vi "Handle INVOCATION.vi"(8 "error in (no error)":errorcluster, 9 "Message Loop Shift Register Data":T1, 10 "Cluster":T8 {"Message Codes" items=["HELLO"=1, "WELCOME"=2, "ABORT"=3, "GOODBYE"=6, "ERROR"=8, "PUBLISH"=16, "PUBLISHED"=17, "SUBSCRIBE"=32, "SUBSCRIBED"=33, "UNSUBSCRIBE"=34, "UNSUBSCRIBED"=35, "EVENT"=36, "CALL"=48, "RESULT"=59, "REGISTER"=64, "REGISTERED"=65, "UNREGISTER"=66, "UNREGISTERED"=67, "INVOCATION"=68, "YIELD"=70]}, 11 "reference":refnum<class "WAMP Client.lvclass">) -> (0 "error out":errorcluster, 3 "reference out":refnum<class "WAMP Client.lvclass">)   [LabVIEW 2020, in "wamplv.lvlib" / "WAMP Client.lvclass"]
uses:
  <userlib>/wamplv/WAMP Client/WAMP Client.lvclass
  <userlib>/wamplv/WAMP Client/TypeDef/WAMP Received Message.ctl
  <userlib>/wamplv/WAMP Message Codes.ctl
  <userlib>/wamplv/WAMP Client/TypeDef/Message Loop Shift Reg Data.ctl
  <userlib>/wamplv/WAMP Client/TypeDef/REGISTER Request Data.ctl
  <userlib>/wamplv/WAMP Client/TypeDef/REGISTERED or ERROR payload.ctl
  <userlib>/wamplv/WAMP Client/TypeDef/WAMP Error Payload.ctl
  <userlib>/wamplv/WAMP Client/TypeDef/INVOCATION payload.ctl
  <userlib>/wamplv/WAMP Client/TypeDef/Publish Requests Map.ctl
  <userlib>/wamplv/WAMP Client/TypeDef/PUBLISH Request Data.ctl
  <userlib>/wamplv/WAMP Client/TypeDef/PUBLISH Result.ctl
  <userlib>/wamplv/WAMP Client/TypeDef/Endpoint Data.ctl
  <userlib>/wamplv/WAMP Client/TypeDef/CALL Request Map.ctl
  <userlib>/wamplv/WAMP Client/TypeDef/CALL Request Data.ctl
  <userlib>/wamplv/WAMP Client/TypeDef/RESULT Payload.ctl
  <userlib>/wamplv/WAMP Client/WAMP Client.lvclass/WAMP Client.ctl
  <vilib>/JDP Science/JSONtext/JSONtext.lvlib
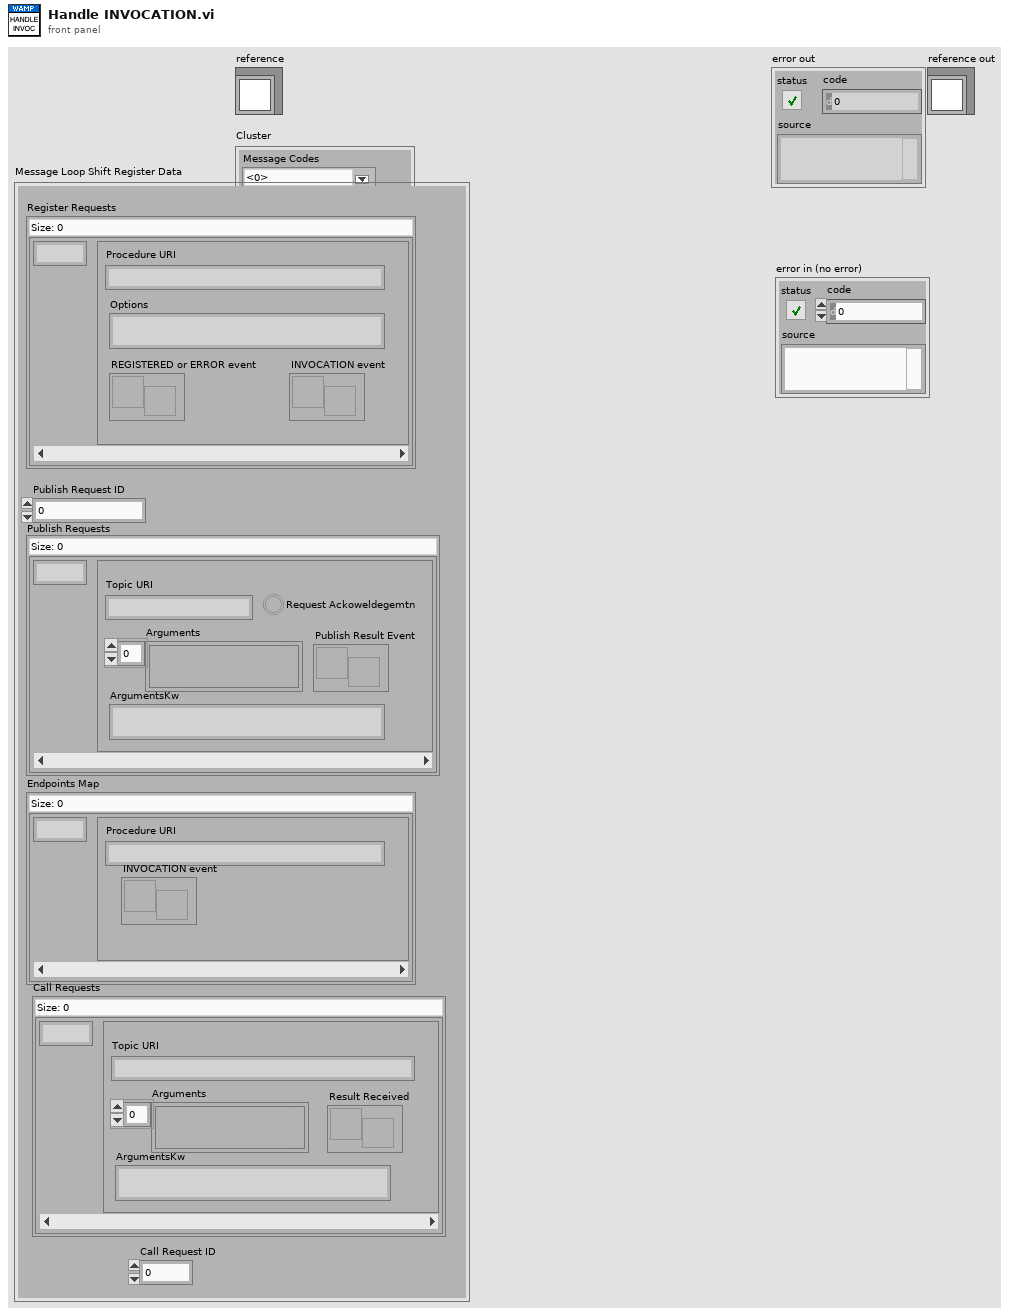
[diagram p1: front panel]
types:
  T1 = typedef "wamplv.lvlib/WAMP Client.lvclass/Message Loop Shift Reg Data.ctl" = cluster{"Register Requests":map{u32, T2}, "Publish Request ID":u32, "Publish Requests":T3, "Endpoints Map":map{u32, T5}, "Call Requests":T6, "Call Request ID":u32}
  T2 = typedef "wamplv.lvlib/WAMP Client.lvclass/REGISTER Request Data.ctl" = cluster{"Procedure URI":string, "Options":string, "REGISTERED or ERROR event":refnum<user-event>, "INVOCATION event":refnum<user-event>}
  T3 = typedef "wamplv.lvlib/WAMP Client.lvclass/Publish Requests Map.ctl" = map{u32, T4}
  T4 = typedef "wamplv.lvlib/WAMP Client.lvclass/PUBLISH Request Data.ctl" = cluster{"Topic URI":string, "Arguments":variant[], "ArgumentsKw":string, "Publish Result Event":refnum<user-event>, "Request Ackoweldegemtn":bool}
  T5 = typedef "wamplv.lvlib/WAMP Client.lvclass/Endpoint Data.ctl" = cluster{"Procedure URI":string, "INVOCATION event":refnum<user-event>}
  T6 = typedef "wamplv.lvlib/WAMP Client.lvclass/CALL Request Map.ctl" = map{u32, T7}
  T7 = typedef "wamplv.lvlib/WAMP Client.lvclass/CALL Request Data.ctl" = cluster{"Topic URI":string, "Arguments":variant[], "ArgumentsKw":string, "Result Received":refnum<user-event>}
  T8 = typedef "wamplv.lvlib/WAMP Client.lvclass/WAMP Received Message.ctl" = cluster{"Message JSON":string[], "Message Codes":T9}
  T9 = typedef "wamplv.lvlib/WAMP Client.lvclass/WAMP Message Codes.ctl" = u16
  T10 = typedef "wamplv.lvlib/WAMP Client.lvclass/INVOCATION payload.ctl" = cluster{"Arguments":string[], "ArgumentKw":string, "Procedure URI":string, "Details":string, "Registration ID":u32, "Request ID":u32}
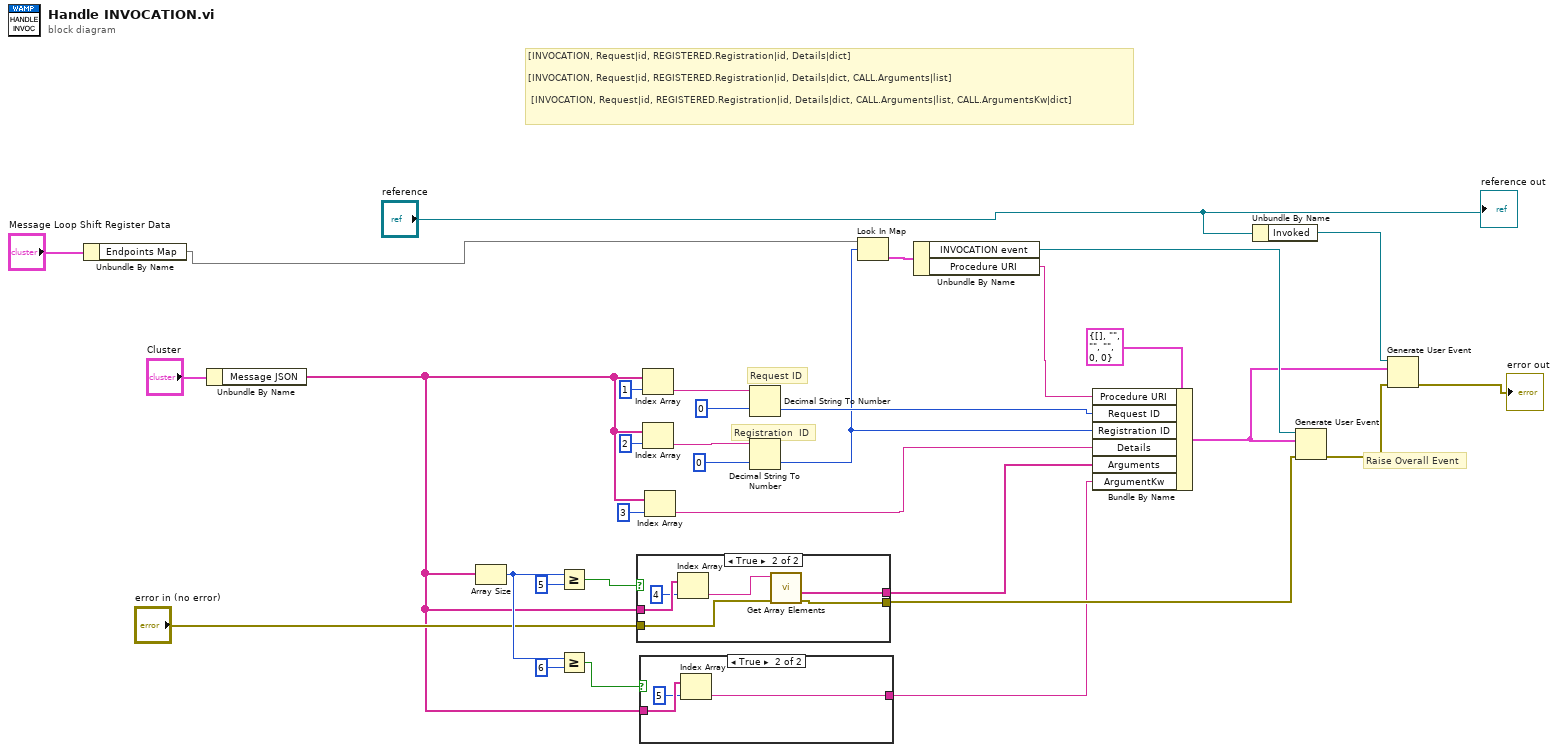
[diagram p0: block diagram]
diagram:
  # "Raise Overall Event"
  # "[INVOCATION, Request|id, REGISTERED.Registration|id, Details|dict]\n\n[INVOCATION, Request|id, REGISTERED.Registration|id, Details|dict, CALL.Arguments|list]\n\n [INVOCATION, Request|id, REGISTERED.Registration|id, Details|dict, CALL.Arguments|list, CALL.ArgumentsKw|dict]"
  # "Registration  ID"
  # "Request ID"
  n1 = Unbundle By Name("Message Loop Shift Register Data") -> ("Endpoints Map"=w10:map{u32, T5})
  n2 = Unbundle By Name("Cluster") -> ("Message JSON"=w4:string[])
  n3 = Array Size(array=w4) -> (size(s)=w22:i32)
  n4 = Greater Or Equal?(x=w22, y=5) -> (x >= y?=w24:bool)
  n5 = Greater Or Equal?(x=w22, y=6) -> (x >= y?=w21:bool)
  n6 = case shown="True" w24 {
    tunnel: w4 -> [_ w38]
    tunnel: [_ w36] -> w6
    tunnel: "error in (no error)" -> [w33 w35]
    tunnel: [w33 w34] -> w19
    frame False {
    }
    frame True {
      n7 = Index Array(array=w38, index=4) -> (element=w39:string)
      n8 = call <vilib>:"Get Array Elements.vi"("error in (no error)"=w35, "JSON"=w39) -> ("error out"=w34:errorcluster, "<JSON>"=w36:string[])  [unwired: 7 in, 1 out]
    }
  }
  n9 = case shown="True" w21 {
    tunnel: w4 -> [_ w42]
    tunnel: [_ w40] -> w5
    frame False {
    }
    frame True {
      n10 = Index Array(array=w42, index=5) -> (element=w40:string)
    }
  }
  n11 = Index Array(array=w4, index=1) -> (element=w31:string)
  n12 = Index Array(array=w4, index=2) -> (element=w32:string)
  n13 = Index Array(array=w4, index=3) -> (element=w7:string)
  n14 = Decimal String To Number(string=w31, default (0L)=u32 0) -> (number=w9:u32)  [unwired: 1 in, 1 out]
  n15 = Decimal String To Number(string=w32, default (0L)=u32 0) -> (number=w8:u32)  [unwired: 1 in, 1 out]
  n16 = Look In Map(map=w10, key=w8) -> (value=w17:T5)  [unwired: 1 in, 1 out]
  n17 = Unbundle By Name(w17) -> ("INVOCATION event"=w2:refnum<user-event>, "Procedure URI"=w16:string)
  n18 = Bundle By Name(cluster=T10 {"Arguments"=[], "ArgumentKw"="", "Procedure URI"="", "Details"="", "Registration ID"=0, "Request ID"=0} ("INVOCATION payload"), "Procedure URI"=w16, "Request ID"=w9, "Registration ID"=w8, "Details"=w7, "Arguments"=w6, "ArgumentKw"=w5) -> (w1:T10)
  n19 = Unbundle By Name("reference") -> ("Invoked"=w14:refnum<user-event>)
  n20 = Generate User Event(user event=w2, event data cluster=w1, error in=w19) -> (error out=w13:errorcluster)  [unwired: 1 in, 1 out]
  n21 = Generate User Event(user event=w14, event data cluster=w1, error in=w13) -> (error out=→"error out":errorcluster)  [unwired: 1 in, 1 out]
  "reference out" <- "reference"
